vi "ReadTexttoArray00.vi"() -> ()   [LabVIEW 2018]
panel:
  out "text":string
  in  "file (use dialog)":path
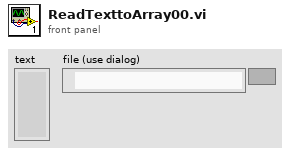
[diagram p1: front panel]
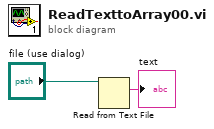
[diagram p0: block diagram]
diagram:
  n1 = Read from Text File(file (use dialog)="file (use dialog)") -> (text=→"text":string)  [unwired: 3 in, 3 out]
